vi "Remove Extraneous Images.vi"(8 "error in (no error)":errorcluster, 11 "XML Path":path) -> (0 "error out":errorcluster)   [LabVIEW 2020, in "Graphical Diff.lvlib"]
uses:
  <vilib>/regexp/Match Regular Expression.xnode
  Graphical Diff.lvlib
panel:
  out "Array 2":string[](array[string])
  out "Deleted Files":path[](array[path])
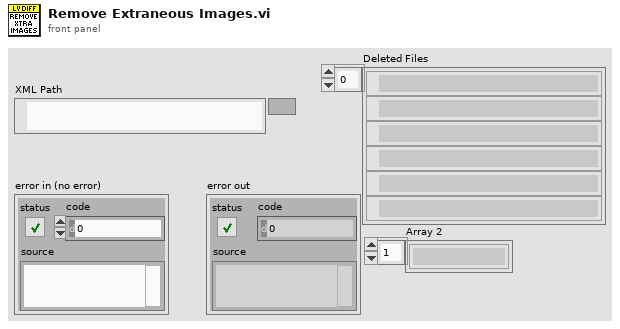
[diagram p1: front panel]
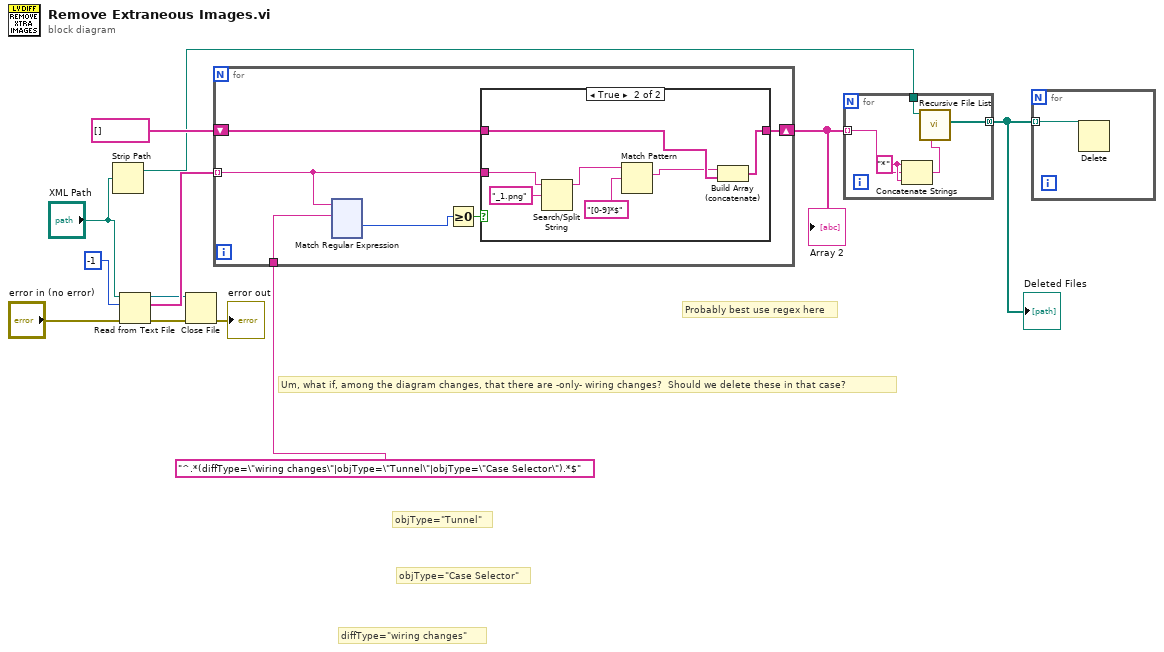
[diagram p0: block diagram]
diagram:
  # "diffType=\"wiring changes\""
  # "objType=\"Case Selector\""
  # "objType=\"Tunnel\""
  # "Probably best use regex here"
  # "Um, what if, among the diagram changes, that there are -only- wiring changes?  Should we delete these in that case?"
  n1 = Strip Path(path="XML Path") -> (stripped path=w3:path)  [unwired: 1 out]
  n2 = Read from Text File(file (use dialog)="XML Path", count=-1, error in="error in (no error)") -> (refnum out=w7:refnum<file>, text=w11:string[], error out=w9:errorcluster)  [unwired: 1 in, 1 out]
  n3 = Close File(refnum=w7, error in=w9) -> (error out=→"error out":errorcluster)  [unwired: 1 out]
  n4 = for {
    tunnel: w11 -> [w14] mode=indexing
    shift-right: [w16] -> w4
    shift-left: string[] [] ("Array 2") -> [w17]
    tunnel: "^.*(diffType=\"wiring changes\"|objType=\"Tunnel\"|objType=\"Case Selector\").*$" ("search string") -> [w13]
    n5 = xnode "Match Regular Expression"("input string"=w14, "regular expression"=w13) -> ("offset past match"=w15:i32)  [unwired: 4 in, 4 out]
    n6 = Greater Or Equal To 0?(x=w15) -> (x >= 0?=w18:bool)
    n7 = case shown="True" w18 {
      tunnel: w17 -> [w133 w138]
      tunnel: [w133 w139] -> w16
      tunnel: w14 -> [_ w137]
      frame False {
      }
      frame True {
        n8 = Search/Split String(string=w137, search string/char (-)="_1.png") -> (substring before match=w136:string)  [unwired: 1 in, 2 out]
        n9 = Match Pattern(string=w136, regular expression="[0-9]*$") -> (match substring=w134:string)  [unwired: 1 in, 3 out]
        n10 = Build Array (concatenate)(w134, w138) -> (w139:string[])
      }
    }
  }
  "Array 2" <- w4
  n11 = for {
    tunnel: w4 -> [w142] mode=indexing
    tunnel: w3 -> [w145]
    tunnel: [w144] -> w2 mode=concatenating
    w143 = "*" ("string")
    n12 = Concatenate Strings(w143, w142, w143) -> (w141:string)
    n13 = call <vilib>:"Recursive File List.vi"("pattern"=w141, "Folder Path"=w145) -> ("All Files in Dir"=w144:path[])  [unwired: 5 in, 4 out]
  }
  "Deleted Files" <- w2
  n14 = for {
    tunnel: w2 -> [w146] mode=indexing
    n15 = Delete(path (use dialog)=w146) -> ()  [unwired: 4 in, 3 out]
  }
